vi "Set Fault.vi"(8 "error in (user fault)":errorcluster={"status"=TRUE, "code"=-66480, "source"=""}, 10 "major fault (F)":bool) -> (0 "error out":errorcluster, 1 "error adding fault":errorcluster)   [LabVIEW 2017]
doc: "Creates a fault. When the <B>major fault</B> input is TRUE, this VI triggers fault mode. Use the <B>code</B> element of the <B>error in (user fault)</B> input cluster to specify the fault code."
uses:
  <resource>/objmgr/ni.var.rc
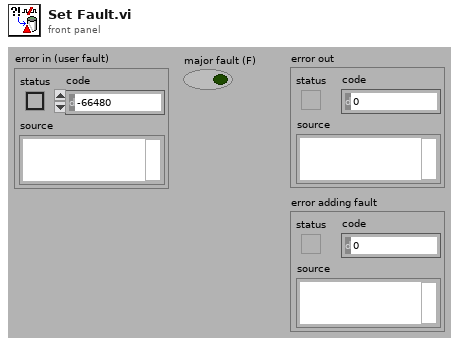
[diagram p1: front panel]
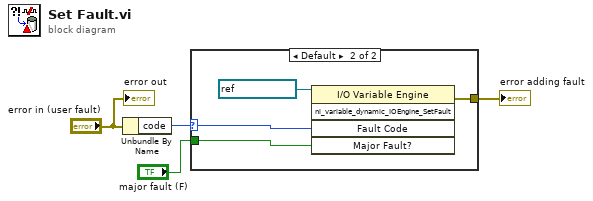
[diagram p0: block diagram]
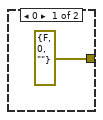
[diagram p2: hidden frame]
diagram:
  n1 = Unbundle By Name("error in (user fault)") -> ("code"=w1:i32)
  n2 = case shown="Default" w1 {
    selector: w1 -> [_ w6]
    tunnel: [errorcluster {"status"=FALSE, "code"=0, "source"=""} ("error out") w7] -> w3
    tunnel: "major fault (F)" -> [_ w8]
    frame 0 {
    }
    frame Default {
      n3 = invoke class="I/O Variable Engine" method="ni_variable_dynamic_IOEngine_SetFault"(reference=refnum<k21> "ni.var.io:/" ("reference out"), "Fault Code"=w6, "Major Fault?"=w8) -> (error out=w7:errorcluster)  [unwired: 2 in, 4 out]
    }
  }
  "error adding fault" <- w3
  "error out" <- "error in (user fault)"
